vi "FIFO_1000ptos_A.vi"(9 "Tamanho da FIFO":i32=1000, 11 "Valor_Entrada":dbl) -> (1 "Array":dbl[](array[numeric]), 3 "Valor_Saída":dbl)   [LabVIEW 2016, in "Biblioteca.lvlib"]
uses:
  Biblioteca.lvlib
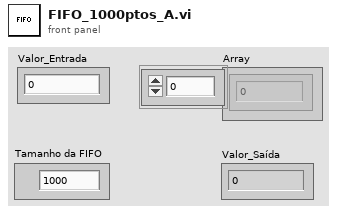
[diagram p1: front panel]
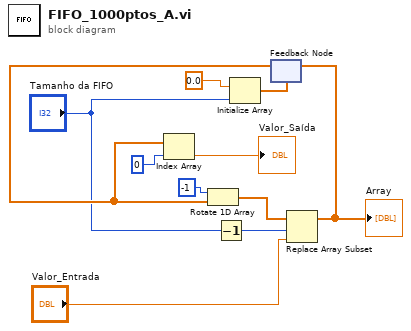
[diagram p0: block diagram]
diagram:
  n1 = Decrement(x="Tamanho da FIFO") -> (x-1=w1:i32)
  n2 = Initialize Array(0.0 ("element"), "Tamanho da FIFO") -> (w9:dbl[])
  n3 = feedback #1(w9) -> (w4:dbl[])
  n4 = Index Array(array=w4, index=0) -> (element=→"Valor_Saída":dbl)
  n5 = Rotate 1D Array(1:w4, 2:-1 ("n")) -> (0:w6:dbl[])
  n6 = Replace Array Subset(array=w6, new element="Valor_Entrada", index=w1) -> (w11:dbl[])
  "Array" <- w11
  n7 = feedback-in #1(w11) -> ()
